vi "Do Draw.vi"(9 "color":u32(colorbox), 10 "picture in":picture, 11 "Circle Message":refnum<class "Circle Message.lvclass">) -> (2 "picture out":picture)   [LabVIEW 2019, in "Draw Messages.lvlib" / "Circle Message.lvclass"]
doc: "Draw whatever the message needs to draw into the picture."
uses:
  Circle Message.lvclass
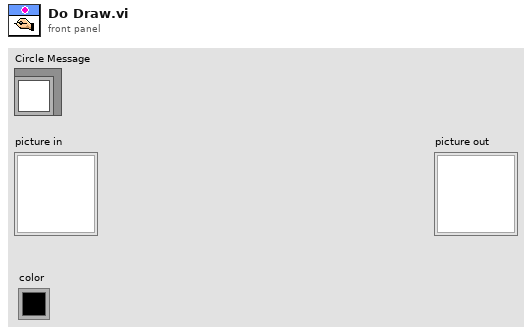
[diagram p1: front panel]
types:
  T1 = cluster{"number: 0 to 1":dbl, "number: 0 to 1":dbl}
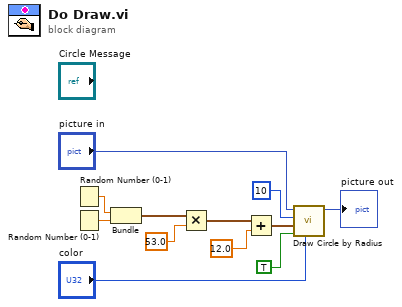
[diagram p0: block diagram]
diagram:
  n1 = Random Number (0-1)() -> (number: 0 to 1=w6:dbl)
  n2 = Random Number (0-1)() -> (number: 0 to 1=w5:dbl)
  n3 = Bundle("number: 0 to 1"=w6, "number: 0 to 1"=w5) -> (w4:T1)  [unwired: 1 in]
  n4 = Multiply(x=w4, y=53.0) -> (x*y=w3:T1)
  n5 = Add(x=w3, y=12.0) -> (x+y=w1:T1)
  n6 = call <vilib>:"Draw Circle by Radius.vi"("color(black)"="color", "fill?(F)"=TRUE, "pixel center"=w1, "radius"=i16 10, "picture"="picture in") -> ("new picture"=→"picture out":picture)  [unwired: 6 in]
